vi "task8(SubVI).vi"(10 "Array":bool[](array[boolean]), 11 "Select number system":T1(ring)) -> (3 "Value:":string)   [LabVIEW 2017]
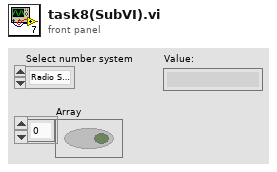
[diagram p1: front panel]
types:
  T1 = enum32{"Radio Selection 1", "Radio Selection 2", "Radio Selection 3", "Radio Selection 4"}
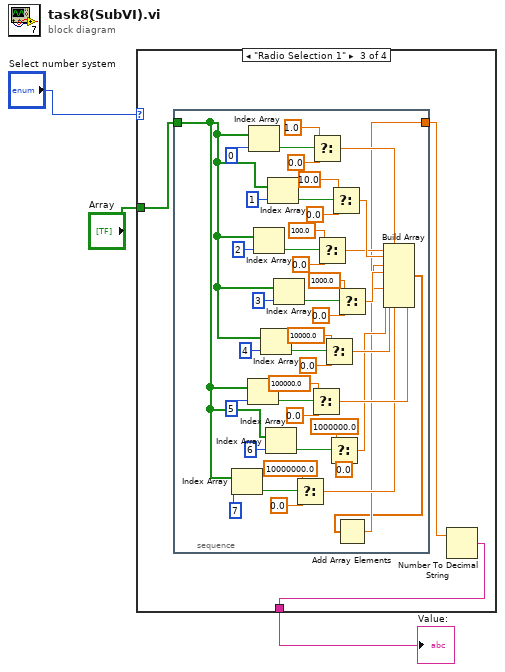
[diagram p0: block diagram]
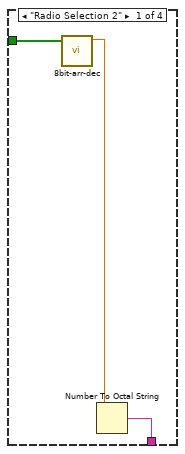
[diagram p2: hidden frame]
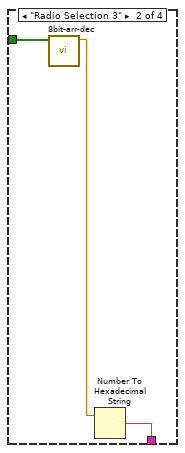
[diagram p3: hidden frame]
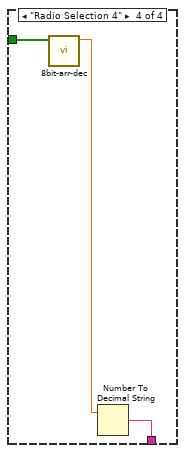
[diagram p4: hidden frame]
diagram:
  n1 = case shown="\"Radio Selection 1\"" "Select number system" {
    tunnel: "Array" -> [w6 w9 w12 w58]
    tunnel: [w4 w8 w11 w57] -> w3
    frame "Radio Selection 2" {
      n2 = call "8bit-arr-dec.vi"("Array"=w6) -> ("f"=w5:dbl)  [unwired: 10 in]
      n3 = Number To Octal String(2:w5) -> (0:w4:string)  [unwired: 1 in]
    }
    frame "Radio Selection 3" {
      n4 = call "8bit-arr-dec.vi"("Array"=w9) -> ("f"=w7:dbl)  [unwired: 10 in]
      n5 = Number To Hexadecimal String(2:w7) -> (0:w8:string)  [unwired: 1 in]
    }
    frame "Radio Selection 1" {
      n6 = stacked-sequence {
        tunnel: [w14] -> w10
        tunnel: w12 -> [w23]
        frame #0 {
          n7 = Index Array(array=w23, index=7) -> (element=w24:bool)
          n8 = Index Array(array=w23, index=5) -> (element=w32:bool)
          n9 = Index Array(array=w23, index=0) -> (element=w52:bool)
          n10 = Index Array(array=w23, index=2) -> (element=w44:bool)
          n11 = Index Array(array=w23, index=4) -> (element=w36:bool)
          n12 = Index Array(array=w23, index=6) -> (element=w28:bool)
          n13 = Index Array(array=w23, index=1) -> (element=w48:bool)
          n14 = Index Array(array=w23, index=3) -> (element=w40:bool)
          n15 = Select(t=10000000.0, s=w24, f=0.0) -> (s? t:f=w15:dbl)
          n16 = Select(t=100000.0, s=w32, f=0.0) -> (s? t:f=w17:dbl)
          n17 = Select(t=1.0, s=w52, f=0.0) -> (s? t:f=w22:dbl)
          n18 = Select(t=100.0, s=w44, f=0.0) -> (s? t:f=w20:dbl)
          n19 = Select(t=10000.0, s=w36, f=0.0) -> (s? t:f=w18:dbl)
          n20 = Select(t=1000000.0, s=w28, f=0.0) -> (s? t:f=w16:dbl)
          n21 = Select(t=10.0, s=w48, f=0.0) -> (s? t:f=w21:dbl)
          n22 = Select(t=1000.0, s=w40, f=0.0) -> (s? t:f=w19:dbl)
          n23 = Build Array(w22, w21, w20, w19, w18, w17, w16, w15) -> (w13:dbl[])
          n24 = Add Array Elements(numeric array=w13) -> (sum=w14:dbl)
        }
      }
      n25 = Number To Decimal String(number=w10) -> (decimal integer string=w11:string)  [unwired: 1 in]
    }
    frame "Radio Selection 4" {
      n26 = call "8bit-arr-dec.vi"("Array"=w58) -> ("f"=w56:dbl)  [unwired: 10 in]
      n27 = Number To Decimal String(number=w56) -> (decimal integer string=w57:string)  [unwired: 1 in]
    }
  }
  "Value:" <- w3
